vi "T_CAN Write data.vi"(8 "error in (no error)":errorcluster, 9 "signal list":refnum<k21>[](array[refnum]), 10 "data":dbl[](array[numeric]) format="%.2f", 11 "CAN SIGNAL":string) -> (0 "error out":errorcluster)   [LabVIEW 2018]
uses:
  <vilib>/xnet/xnet.llb/XNET Create Session (Signal Output Single-point).vi
  <vilib>/xnet/xnet.llb/XNET Write (Signal Single-point).vi
panel:
  out "session out 2":refnum<k21>
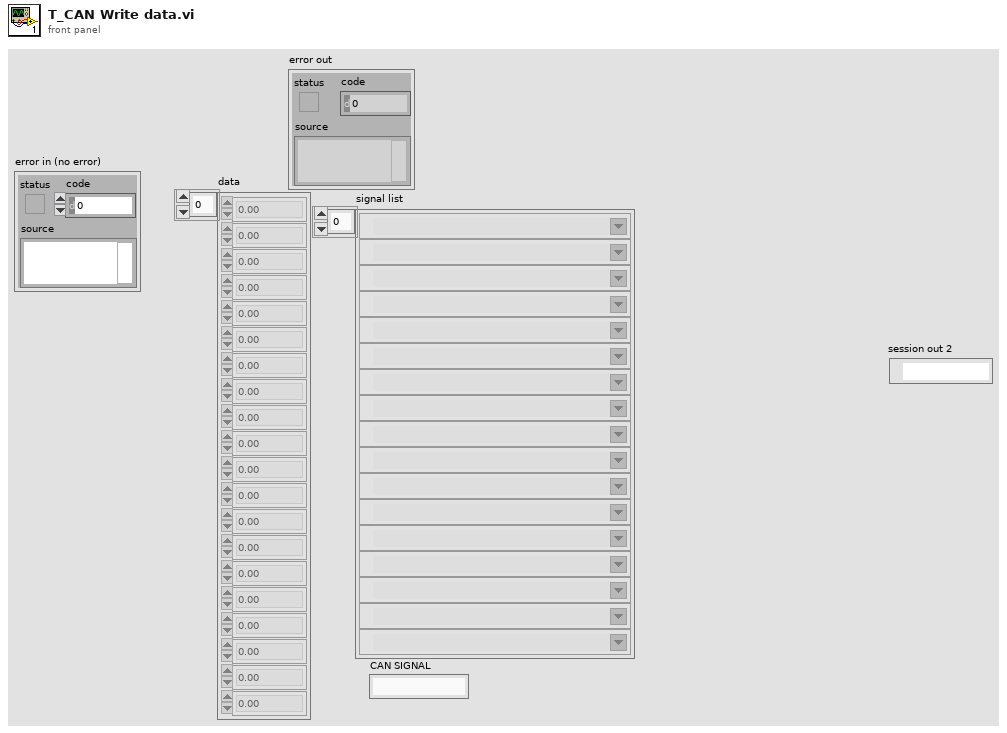
[diagram p1: front panel]
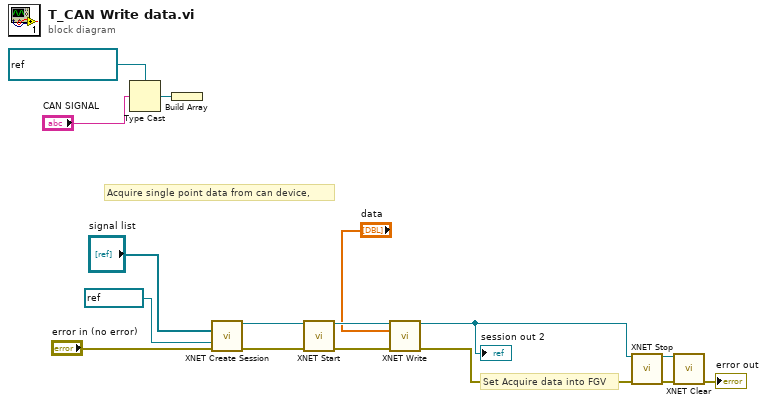
[diagram p0: block diagram]
diagram:
  # "Set Acquire data into FGV"
  # "Acquire single point data from can device,"
  n1 = Type Cast(type=refnum<k21> "EngineOilPrLamp\nTEST" ("XNET Signal"), x="CAN SIGNAL") -> (*(type *) &x=w7:refnum<k21>)
  n2 = Build Array(w7) -> ()  [unwired: 1 out]
  n3 = call-poly <vilib>:"XNET Create Session.vi"("signal list"="signal list", "interface"=refnum<k21> "CAN1" ("Select Interface"), "error in (no error)"="error in (no error)") -> ("session out"=w14:refnum<k21>, "error out"=w15:errorcluster)  [unwired: 11 out]
  n4 = call <vilib>:"XNET Start.vi"("session in"=w14, "error in (no error)"=w15) -> ("session out"=w12:refnum<k21>, "error out"=w11:errorcluster)  [unwired: 12 in]
  n5 = call-poly <vilib>:"XNET Write.vi"("session in"=w12, "data"="data", "error in (no error)"=w11) -> ("session out"=w9:refnum<k21>, "error out"=w10:errorcluster)  [unwired: 11 in]
  "session out 2" <- w9
  n6 = call <vilib>:"XNET Stop.vi"("session in"=w9, "error in (no error)"=w10) -> ("session out"=w3:refnum<k21>, "error out"=w2:errorcluster)  [unwired: 12 in]
  n7 = call <vilib>:"XNET Clear.vi"("session in"=w3, "error in (no error)"=w2) -> ("error out"=→"error out":errorcluster)  [unwired: 13 in]
